vi "Time-Frequency Resolution.vi"() -> ()   [LabVIEW 2023]
doc: "This example shows the window effect of the STFT spectrogram. The STFT spectrogram usually is sufficient for most applications, but it typically provides a coarse time-frequency resolution as a result of window effects that the window type and the window length determine. A narrow window results in a fine time resolution but a coarse frequency resolution because narrow windows have a short time duration but a wide bandwidth. A wide window results in a fine frequency resolution but a coarse time resolution because wide windows have a long time duration but a narrow frequency bandwidth. You cannot obtain a fine time resolution and a fine frequency resolution simultaneously using the STFT spectrogram.\n\n<b>Instructions:</b>\n1) Run this VI.\n2) Slide the value of Window Length to observe how the window length affects the time-frequency resolution of the STFT spectrogram."
uses:
  <vilib>/addons/Time Frequency Analysis/typedefs.llb/TFA Data.ctl
  <vilib>/Analysis/4window.llb/windowTd.ctl
  <vilib>/Analysis/0measdsp.llb/Scaled Time Domain Window (DBL).vi
  <vilib>/addons/Time Frequency Analysis/Spectrogram.llb/TFA STFT Spectrogram (Waveform).vi
  <vilib>/addons/Time Frequency Analysis/_control.llb/TFA Configure Spectrogram Indicator (Predefined Color Table).vi
  <vilib>/addons/_Advanced Signal Processing/NI_AdvSigProcTFA.lvlib
  <vilib>/Analysis/NI_AALPro.lvlib
panel:
  out "aspt-left-top":bool
  out "Signal":waveform(dbl)(graph)
  in  "stop":bool
  in  "Window length":i32(slide)=57 scale=10.0..256.0
  out "Sliding Window":dbl[](graph)
  out "STFT Spectrogram":dbl[][](graph)
  # "Overview: Shows the window effect of the STFT spectrogram.\nRequirements: LabVIEW Full Development System, Advanced Signal Processing Toolkit\nInstructions: \n1. Run this VI.\n2. Slide the value of Window Length to observe how the window length affects the time-frequency resolution of the STFT spectrogram.\n3. Click Stop to stop the VI."
  # "Low"
  # "High"
  # "Frequency Resolution"
  # "Time Resolution"
  # "Low"
  # "High"
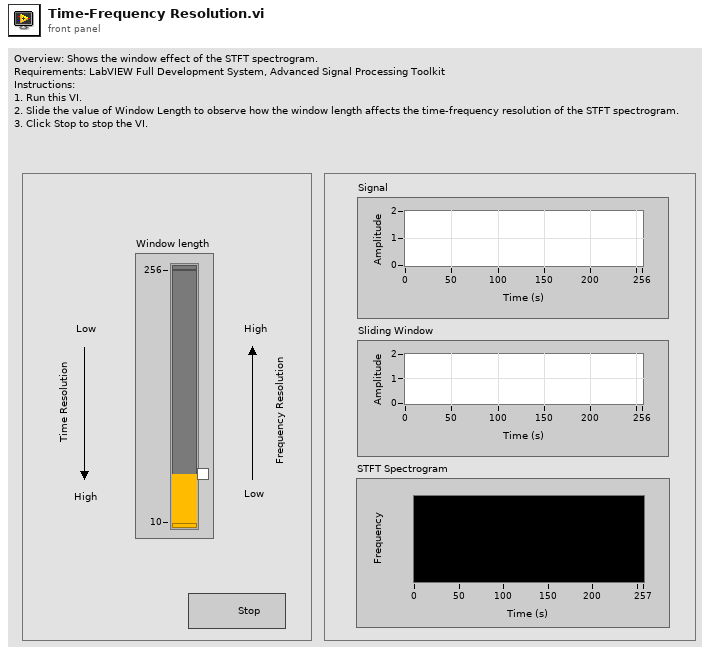
[diagram p1: front panel]
types:
  T1 = typedef "NI_AALPro.lvlib/windowTd.ctl" = u32
  T2 = typedef "NI_AdvSigProcTFA.lvlib/TFA Data.ctl" = u16
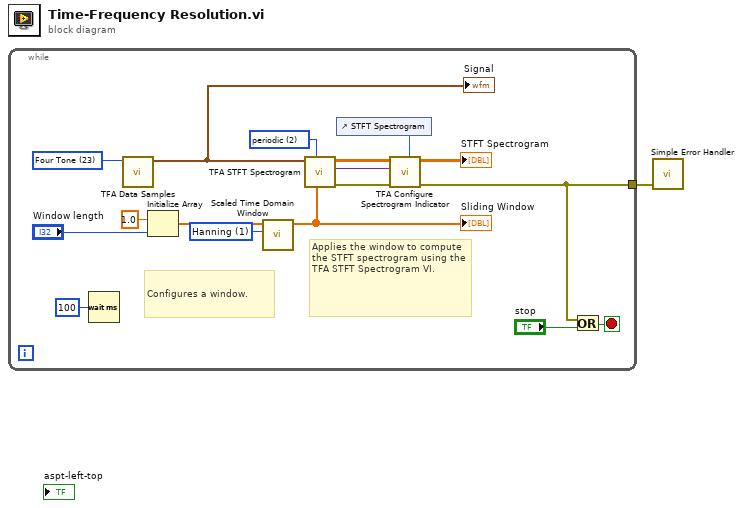
[diagram p0: block diagram]
diagram:
  n1 = while {
    tunnel: [w2] -> w1
    stop <- w3 stop-if-true
    w6 = T1 1 items=["Rectangle"=0, "Hanning"=1, "Hamming"=2, "Blackman-Harris"=3, "Exact Blackman"=4, "Blackman"=5, "Flat Top"=6, "4 Term B-Harris "=7, "7 Term B-Harris"=8, "Low Sidelobe"=9, "Blackman Nuttall"=11, "Triangle"=30, "Bartlett-Hanning"=31, "Bohman"=32, "Parzen"=33, "Welch"=34, "Kaiser"=60, "Dolph-Chebyshev"=61, "Gaussian"=62] ("window")
    w7 = T2 23 items=["PC Fan"=0, "Noisy Chirps"=1, "TDR 1"=2, "TDR 2"=3, "Liquefaction"=4, "Liquefaction Free"=5, "Aneurysm"=6, "Bat"=7, "RF"=8, "Two Gaussian"=9, "Three Gaussian"=10, "Chirp"=11, "Gaussian Chirp"=12, "Cross Chirp"=13, "Doppler"=14, "HOP"=15, "TF Sine"=16, "Three Tone"=17, "Four Tone"=23, "Blood Flow Doppler (phase a)"=20, "Blood Flow Doppler (phase b)"=21, "Heart sound"=22, "-"=18, "Random Noise"=19] ("data")
    w14 = u16 2 items=["zero padding", "symmetric", "periodic"] ("extension")
    # "Applies the window to compute the STFT spectrogram using the TFA STFT Spectrogram VI."
    # "Configures a window."
    n2 = Wait (ms)(milliseconds to wait=u32 100 ("millisecond multiple")) -> ()  [unwired: 1 out]
    n3 = call <vilib>:"TFA Data Samples.vi"("data"=w7) -> ("signal"=w8:waveform(dbl))  [unwired: 10 out]
    "Signal" <- w8
    n4 = Initialize Array(1.0 ("element"), "Window length") -> (w16:dbl[])
    n5 = call-poly <vilib>:"Scaled Time Domain Window.vi"("window"=w6, "X"=w16) -> ("Windowed X"=w15:dbl[])  [unwired: 1 in, 8 out]
    "Sliding Window" <- w15
    n6 = call-poly <vilib>:"TFA STFT Spectrogram.vi"("user defined window"=w15, "extension"=w14, "signal"=w8) -> ("error out"=w5:errorcluster, "scale info"=w12:variant, "spectrogram"=w13:dbl[][])  [unwired: 3 in, 3 out]
    n7 = control-ref of="STFT Spectrogram"() -> (w10:refnum<vi>)
    n8 = call-poly <vilib>:"TFA Configure Spectrogram Indicator.vi"("reference of TF spectrogram indicator"=w10, "error in (no error)"=w5, "scale info"=w12, "spectrogram"=w13) -> ("error out"=w2:errorcluster, "TF spectrogram indicator"=→"STFT Spectrogram":dbl[][])  [unwired: 3 in, 3 out]
    n9 = Or(x=w2, y="stop") -> (x .or. y?=w3:bool)
  }
  n10 = call <vilib>:"Simple Error Handler.vi"("error in (no error)"=w1) -> ()  [unwired: 4 in, 5 out]
